vi "Cleanup Protection Frames.vi"(11 "Frames":T1[](array[typedef]) {"Protection Configurations"."CRC Channels"."Data Type" items=["Signed", "Unsigned", "IEEE Float"]}) -> (0 "error out":errorcluster)   [LabVIEW 2023, in "Protection and Counter Support Engine.lvlib"]
uses:
  Protection and Counter Support Engine.lvlib
  Types/RT Frame Settings.ctl
  Shared/Types/Exported Frame Type.ctl
  Types/RT Protection Configuration.ctl
  Shared/Types/Protection Type.ctl
  Shared/Types/XNET Signal Configuration.ctl
  Shared/Types/Exported Counter Settings.ctl
  Shared/Types/Exported Event Trigger Type.ctl
  Shared/Protection and Counter Support Shared.lvlib
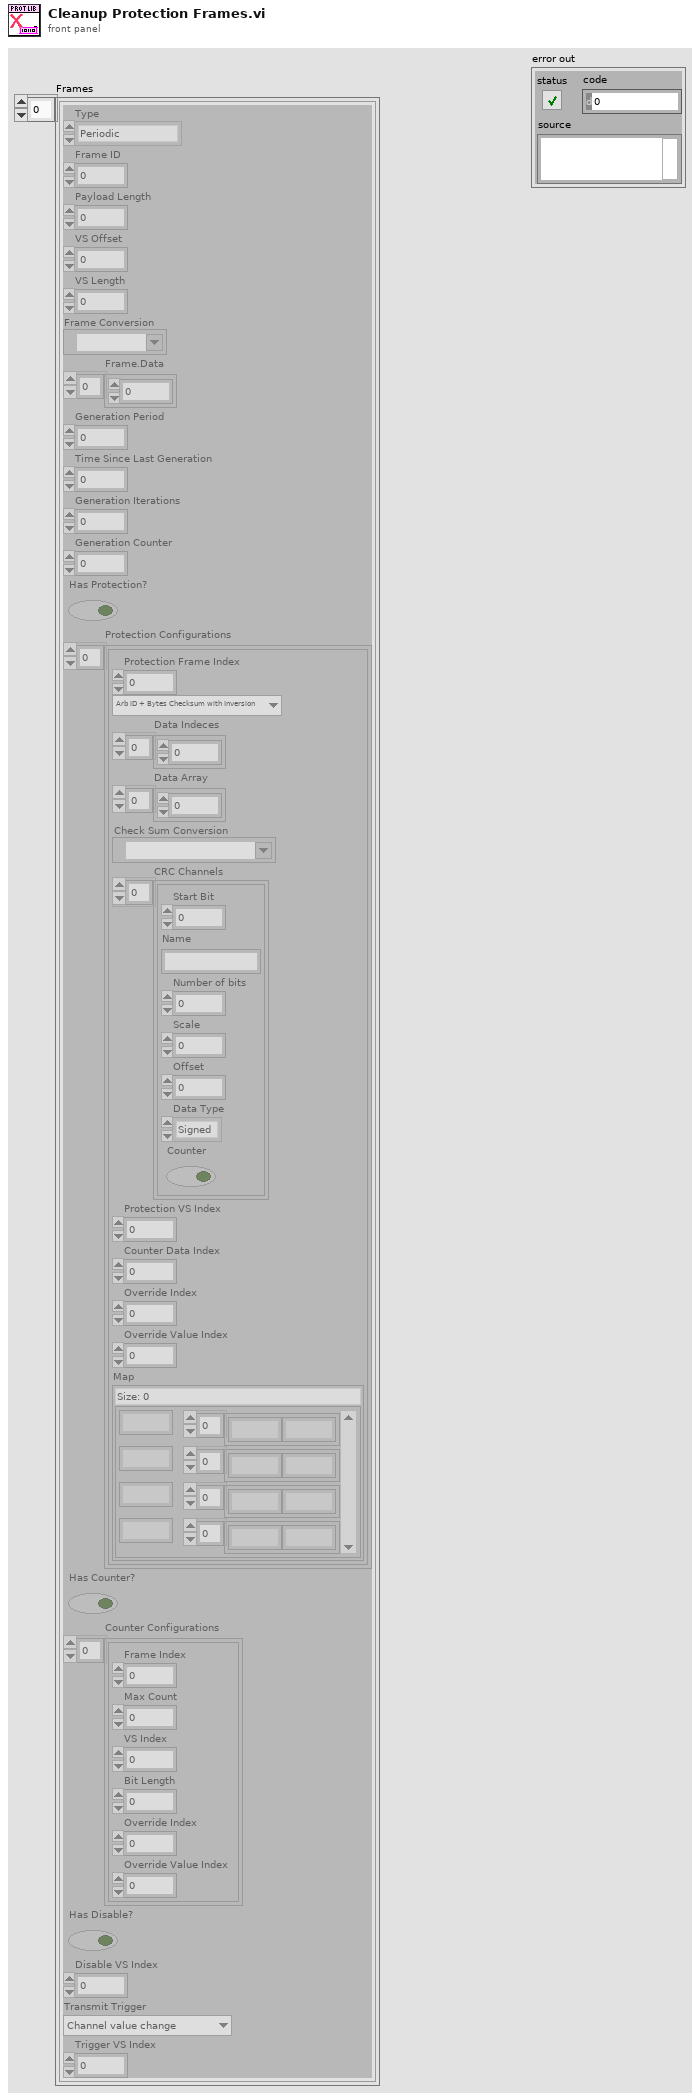
[diagram p1: front panel]
types:
  T1 = typedef "Protection and Counter Support Engine.lvlib/RT Frame Settings.ctl" = cluster{"Type":T2, "Frame ID":u32, "Payload Length":u32, "VS Offset":i32, "VS Length":i32, "Frame Conversion":refnum<k21>, "Frame.Data":dbl[], "Generation Period":u32, "Time Since Last Generation":u32, "Generation Iterations":u32, "Generation Counter":u32, "Has Protection?":bool, "Protection Configurations":T3[], "Has Counter?":bool, "Counter Configurations":T6[], "Has Disable?":bool, "Disable VS Index":i32, "Transmit Trigger":T7, "Trigger VS Index":i32}
  T2 = typedef "Protection and Counter Support Shared.lvlib/Exported Frame Type.ctl" = enum16{"Periodic", "Event", "Periodic/Event"}
  T3 = typedef "Protection and Counter Support Engine.lvlib/RT Protection Configuration.ctl" = cluster{"Protection Frame Index":i32, "Protection Type":T4, "Data Indeces":i32[], "Data Array":dbl[], "Check Sum Conversion":refnum<k21>, "CRC Channels":T5[], "Protection VS Index":i32, "Counter Data Index":i32, "Override Index":i32, "Override Value Index":i32, "Map":map{i32, u8[]}}
  T4 = typedef "Protection and Counter Support Shared.lvlib/Protection Type.ctl" = enum16{"Arb ID + Bytes Checksum with Inversion", "Arb ID + Bytes CRC with Inversion", "Reversed Raw Signal Checksum with Inversion", "Concatenated Two's Compliment", "LP_CRC8", "LP_Checksum", "LP_CRC8_MRS"}
  T5 = typedef "Protection and Counter Support Shared.lvlib/XNET Signal Configuration.ctl" = cluster{"Start Bit":i32, "Name":string, "Number of bits":i32, "Scale":dbl, "Offset":dbl, "Data Type":u32, "Counter":bool}
  T6 = typedef "Protection and Counter Support Shared.lvlib/Exported Counter Settings.ctl" = cluster{"Frame Index":i32, "Max Count":dbl, "VS Index":i32, "Bit Length":i64, "Override Index":i32, "Override Value Index":i32}
  T7 = typedef "Protection and Counter Support Shared.lvlib/Exported Event Trigger Type.ctl" = enum16{"Channel value change", "Trigger channel (not zero)", "Channel value change or trigger channel (not zero)", "Trigger channel (any value change)", "Channel value change or trigger channel (any value change)"}
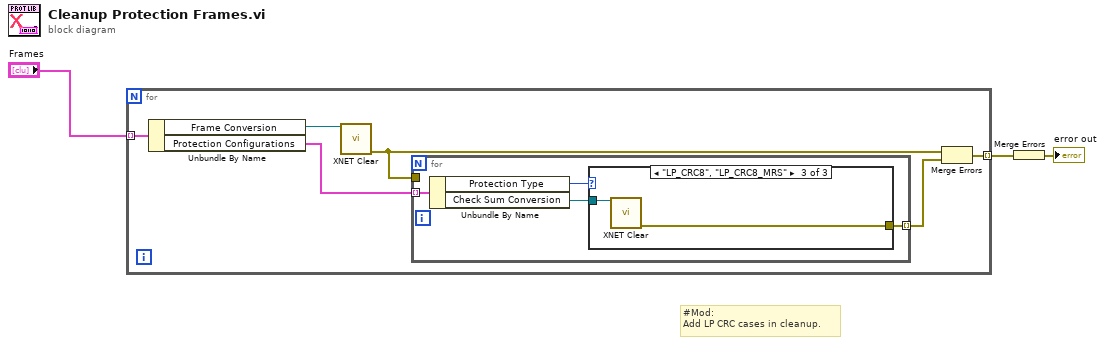
[diagram p0: block diagram]
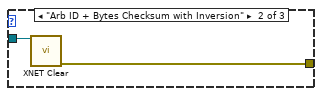
[diagram p3: hidden frame]
diagram:
  # "#Mod:\nAdd LP CRC cases in cleanup."
  n1 = for {
    tunnel: "Frames" -> [w9] mode=indexing
    tunnel: [w4] -> w2 mode=indexing
    n2 = Unbundle By Name(w9) -> ("Frame Conversion"=w8:refnum<k21>, "Protection Configurations"=w7:T3[])
    n3 = call <vilib>:"XNET Clear.vi"("session in"=w8) -> ("error out"=w6:errorcluster)  [unwired: 14 in]
    n4 = for {
      tunnel: w7 -> [w13] mode=indexing
      tunnel: [w11] -> w5 mode=indexing
      tunnel: w6 -> [_]
      n5 = Unbundle By Name(w13) -> ("Protection Type"=w10:T4, "Check Sum Conversion"=w12:refnum<k21>)
      n6 = case shown="\"LP_CRC8\", \"LP_CRC8_MRS\"" w10 {
        tunnel: w12 -> [_ w15 w17]
        tunnel: [_ w14 w16] -> w11
        frame Default {
        }
        frame "Arb ID + Bytes Checksum with Inversion" {
          n7 = call <vilib>:"XNET Clear.vi"("session in"=w15) -> ("error out"=w14:errorcluster)  [unwired: 14 in]
        }
        frame "LP_CRC8", "LP_CRC8_MRS" {
          n8 = call <vilib>:"XNET Clear.vi"("session in"=w17) -> ("error out"=w16:errorcluster)  [unwired: 14 in]
        }
      }
    }
    n9 = Merge Errors(w6, w5) -> (w4:errorcluster)
  }
  n10 = Merge Errors(w2) -> (→"error out":errorcluster)
